vi "Abort.vi"(0 "eye scan single point":refnum<class "niHighSpeedSerial Eye Scan Single Point v1 Host.lvclass">, 11 "error in":errorcluster) -> (4 "eye scan single point out":refnum<class "niHighSpeedSerial Eye Scan Single Point v1 Host.lvclass">, 15 "error out":errorcluster)   [LabVIEW 2014, in "niHighSpeedSerial Eye Scan Single Point v1 Host.lvclass"]
doc: "Stops the Eye Scan engine from running on the channel.\n\n<B>Input Parameters</B>\n\n<B>eye scan single point</B> takes in a reference to your session from the previous VI.\n\n<B>error in</B> describes error conditions that occur before this node runs. This input provides standard 'error in' functionality.\n\n<B>Output Parameters</B>\n\n<B>eye scan single point out</B> passes a reference to your session to the next VI.\n\n<B>error out</B> contains error information. This output provides standard 'error out' functionality."
uses:
  <instrlib>/niHighSpeedSerial/Eye Scan/v1/Host/Impl/Single Point/niHighSpeedSerial Eye Scan Single Point v1 Host.lvclass
  <instrlib>/niHighSpeedSerial/Eye Scan/v1/Host/Impl/Single Point/niHighSpeedSerial Eye Scan Single Point v1 Host.lvclass/niHighSpeedSerial Eye Scan Single Point v1 Host.ctl
  <instrlib>/niHighSpeedSerial/Eye Scan/v1/Host/Impl/Single Point/Private/Channel Measure State.ctl
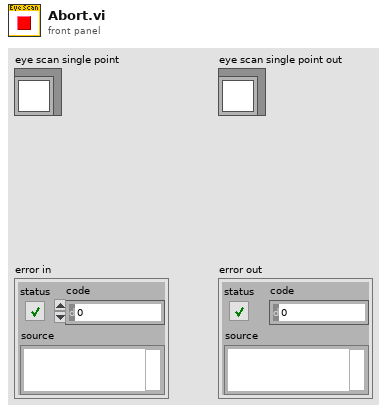
[diagram p1: front panel]
types:
  T1 = typedef "niHighSpeedSerial Eye Scan Single Point v1 Host.lvclass/Channel Measure State.ctl" = enum16{"Uninitialized", "Initialized", "Ready", "Request", "Wait", "Read", "Process", "Finished"}
  T2 = typedef "niHighSpeedSerial Eye Scan Single Point v1 Host.lvclass/Private Data.ctl" = cluster{"GTX2_CHANNEL register map":refnum<class "GTX2_CHANNEL Register Map.lvclass">, "instruction target":refnum<class "niInstr Instruction Target v1 Host.lvclass">, "channel measure state":T1, "in DFE mode?":bool, "prescale":u8, "receiver data width":T3, "active point":T4, "ut sign":T5, "positive counts":T6, "negative counts":T6}
  T3 = typedef "niHighSpeedSerial Eye Scan Common v1 Host.lvlib/Data Width.ctl" = enum16{"16 Bit", "20 Bit", "32 Bit", "40 Bit"}
  T4 = typedef "niHighSpeedSerial Eye Scan Common v1 Host.lvlib/Point Offsets.ctl" = cluster{"horizontal offset":i16, "vertical offset":i8}
  T5 = typedef "GTX2_CHANNEL v1 Host.lvlib/ESVertOffsetSign.ctl" = enum8{"Positive", "Negative"}
  T6 = typedef "niHighSpeedSerial Eye Scan Single Point v1 Host.lvclass/Counts.ctl" = cluster{"sample count":u64, "error count":u16}
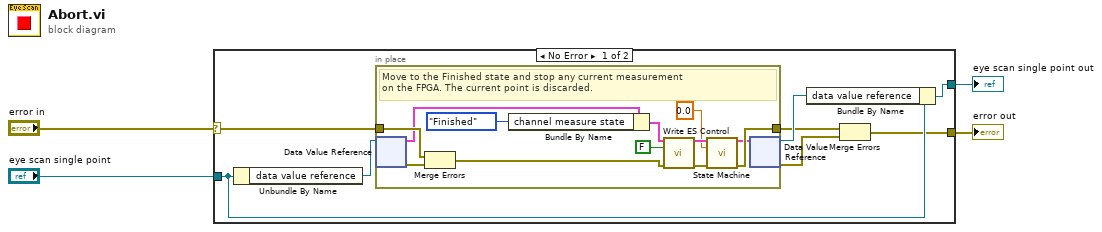
[diagram p0: block diagram]
diagram:
  n1 = case shown="No Error" "error in" {
    selector: "error in" -> [w8 w26]
    tunnel: [w5 w26] -> w3
    tunnel: [w9 w25] -> w2
    tunnel: "eye scan single point" -> [w11 w25]
    frame No Error {
      n2 = Unbundle By Name(w11) -> ("data value reference"=w12:refnum<data-value>)
      n3 = in-place {
        in-place-border: w8 -> [w24]
        in-place-border: [w16] -> w6
        # "Move to the Finished state and stop any current measurement\non the FPGA. The current point is discarded."
        n4 = in-place-dvr #1(w12) -> (w22:T2, w23:errorcluster)
        n5 = Merge Errors(w24, w23) -> (w19:errorcluster)
        n6 = Bundle By Name(cluster=w22, "channel measure state"=Channel_Measure_State."Finished" ("Channel Measure State")) -> (w20:T2)
        n7 = call <instrlib>:"Write ES Control.vi"("private data"=w20, "run?"=FALSE ("Run?"), "error in"=w19) -> ("private data out"=w15:T2, "error out"=w17:errorcluster)  [unwired: 11 in]
        n8 = call <instrlib>:"State Machine.vi"("private data"=w15, "timeout (100 ms)"=0.0 ("Timeout (100 ms)"), "error in"=w17) -> ("private data out"=w14:T2, "error out"=w16:errorcluster)  [unwired: 6 in, 5 out]
        n9 = in-place-dvr #1(w14) -> (w10:refnum<data-value>, w7:errorcluster)
      }
      n10 = Bundle By Name(cluster=w11, "data value reference"=w10) -> (w9:refnum<class "niHighSpeedSerial Eye Scan Single Point v1 Host.lvclass">)
      n11 = Merge Errors(w6, w7) -> (w5:errorcluster)
    }
    frame Error {
    }
  }
  "eye scan single point out" <- w2
  "error out" <- w3
